vi "AlliGator Formula Interpreter.vi"(8 "error in (no error)":errorcluster, 11 "Original Formula":string) -> (0 "error out":errorcluster, 1 "Variable Names":cluster{"Array of Names":string[]}, 2 "Variable Indices":cluster{"Array of Indices":i32[]}, 3 "Interpreted Formula":string, 4 "Unused Flag":bool)   [LabVIEW 2021, in "AlliGator Phasor Plot.lvlib"]
doc: "Replaces user quantities by definitions in the provided formula."
uses:
  AlliGator Phasor Plot.lvlib
  Formula/Formula.lvlib
panel:
  # "see the AlliGator License on the block diagram (Ctrl+E or Window:Show Block Diagram)"
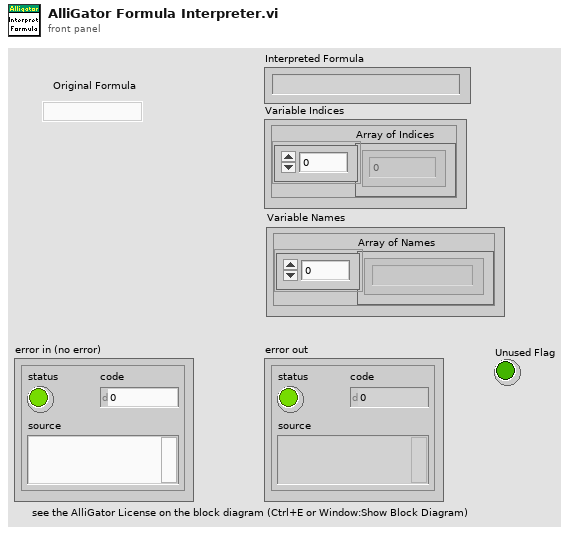
[diagram p1: front panel]
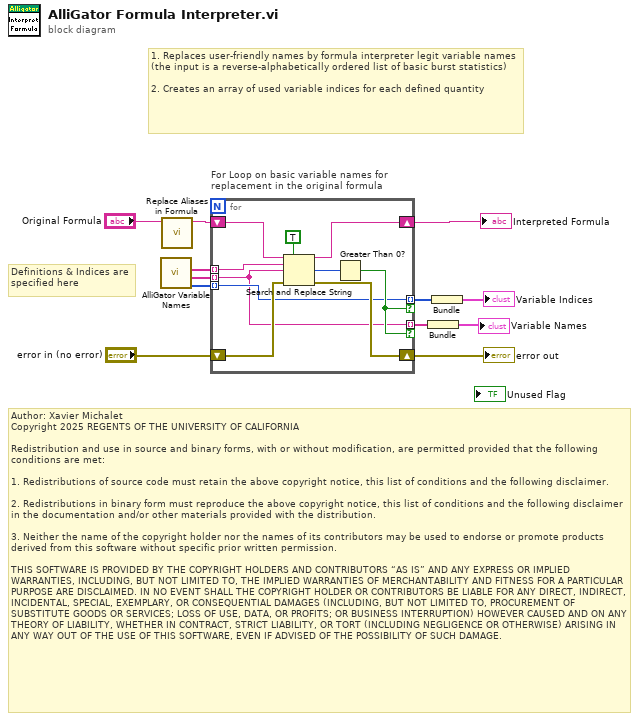
[diagram p0: block diagram]
diagram:
  # "Author: Xavier Michalet\nCopyright 2025 REGENTS OF THE UNIVERSITY OF CALIFORNIA\n\nRedistribution and use in source and binary forms, with or without modification, are permitted provided that the following conditions are met:\n\n1. Redistributions of source code must retain the above copyright notice, this list of conditions and the following disclaimer.\n\n2. Redistributions in binary form must reproduce the above copyright notice, this list of conditions and the following disclaimer in the documentation and/or other materials provided with the distribution.\n\n3. Neither the name of the copyright holder nor the names of its contributors may be used to endorse or promote products derived from this software without specific prior written permission.\n\nTHIS SOFTWARE IS PROVIDED BY THE COPYRIGHT HOLDERS AND CONTRIBUTORS “AS IS” AND ANY EXPRESS OR IMPLIED WARRANTIES, INCLUDING, BUT NOT LIMITED TO, THE IMPLIED WARRANTIES OF MERCHANTABILITY AND FITNESS FOR A PARTICULAR PURPOSE ARE DISCLAIMED. IN NO EVENT SHALL THE COPYRIGHT HOLDER OR CONTRIBUTORS BE LIABLE FOR ANY DIRECT, INDIRECT, INCIDENTAL, SPECIAL, EXEMPLARY, OR CONSEQUENTIAL DAMAGES (INCLUDING, BUT NOT LIMITED TO, PROCUREMENT OF SUBSTITUTE GOODS OR SERVICES; LOSS OF USE, DATA, OR PROFITS; OR BUSINESS INTERRUPTION) HOWEVER CAUSED AND ON ANY THEORY OF LIABILITY, WHETHER IN CONTRACT, STRICT LIABILITY, OR TORT (INCLUDING NEGLIGENCE OR OTHERWISE) ARISING IN ANY WAY OUT OF THE USE OF THIS SOFTWARE, EVEN IF ADVISED OF THE POSSIBILITY OF SUCH DAMAGE."
  # "Definitions & Indices are specified here"
  # "1. Replaces user-friendly names by formula interpreter legit variable names (the input is a reverse-alphabetically ordered list of basic burst statistics)\n\n2. Creates an array of used variable indices for each defined quantity"
  n1 = call "AlliGator Variable Names.vi"() -> ("Sorted Index Array"=w1:i32[], "Sorted Variable Internal Names"=w2:string[], "Sorted Basic Variable Names"=w3:string[])  [unwired: 5 in, 1 out]
  n2 = call "Replace Aliases in Formula.vi"("Definition in"="Original Formula") -> ("Expanded Definition out"=w4:string)  [unwired: 10 in]
  n3 = for "For Loop on basic variable names for replacement in the original formula" {
    tunnel: w3 -> [w21] mode=indexing
    shift-right: [w20] -> w8
    shift-left: w4 -> [w22]
    shift-right: [w18] -> w10
    shift-left: "error in (no error)" -> [w19]
    tunnel: [w14] -> w11 mode=indexing if=w15
    tunnel: [w13] -> w7 mode=indexing if=w15
    tunnel: w2 -> [w13] mode=indexing
    tunnel: w1 -> [w14] mode=indexing
    n4 = Search and Replace String(replace all?=TRUE ("replace all? (F)"), input string=w22, search string=w21, replace string=w13, error in=w19) -> (result string=w20:string, number of replacements=w17:i32, error out=w18:errorcluster)  [unwired: 3 in, 1 out]
    n5 = Greater Than 0?(x=w17) -> (x > 0?=w15:bool)
  }
  "error out" <- w10
  "Interpreted Formula" <- w8
  n6 = Bundle(w7) -> (→"Variable Names":cluster{string[]})  [unwired: 1 in]
  n7 = Bundle(w11) -> (→"Variable Indices":cluster{i32[]})  [unwired: 1 in]
